vi "Savelot.vi"(5 "Type":string, 7 "Wafer ID":string, 8 "error in (no error)":errorcluster, 11 "LotData in":refnum<class "LotData.lvclass">) -> (0 "error out":errorcluster, 3 "LotData out":refnum<class "LotData.lvclass">)   [LabVIEW 2012, in "LotData.lvclass"]
uses:
  LotData.lvclass
  LotData.lvclass/LotData.ctl
  <vilib>/Utility/file.llb/Read From Spreadsheet File (string).vi
  <vilib>/Utility/file.llb/Write To Spreadsheet File (string).vi
  <vilib>/Utility/file.llb/Write To Spreadsheet File (DBL).vi
panel:
  out "Array":string[][](array[string])
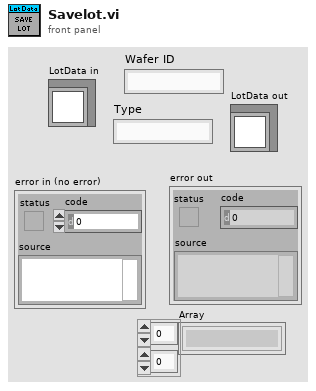
[diagram p1: front panel]
types:
  T1 = cluster{"Area":string, "Wavelength":dbl[], "EL Spectrum":dbl[]}[]
  T2 = typedef "TestData.ctl" = cluster{"20mA Data":cluster{"Area":string, "Current,mA":dbl, "Power":dbl, "WL":dbl, "Voltage":dbl, "Knee Current":dbl, "Reverse":dbl}, "50mA Data":cluster{"Area":string, "Current,mA":dbl, "Power":dbl, "WL":dbl, "Voltage":dbl}}
  T3 = typedef "WaferTable.ctl" = string[][]
  T4 = cluster{"Area":string, "Current,mA":dbl, "Power":dbl, "WL":dbl, "Voltage":dbl, "Knee Current":dbl, "Reverse":dbl}
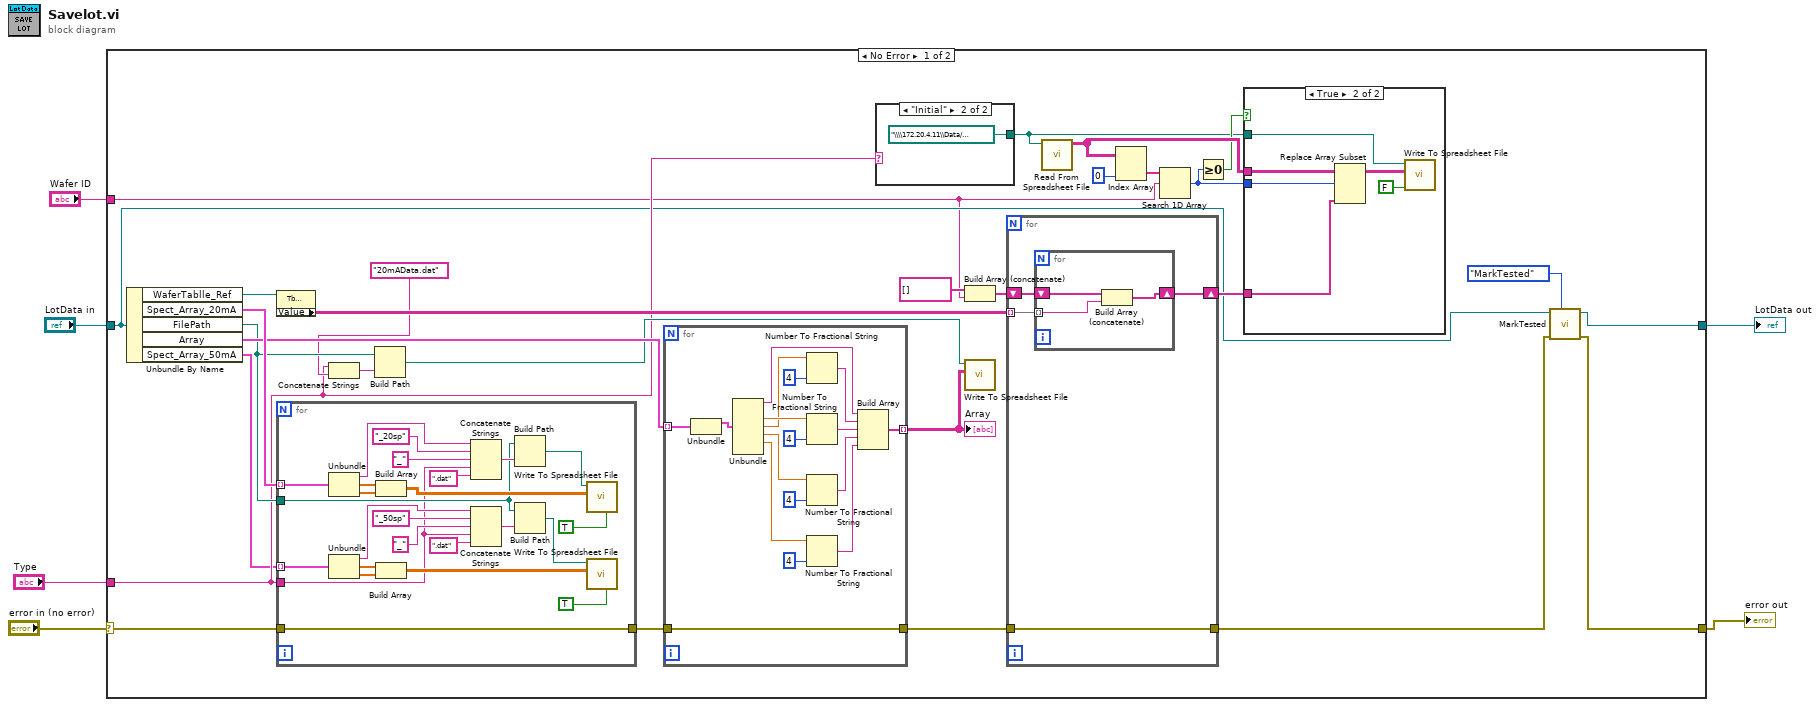
[diagram p0: block diagram]
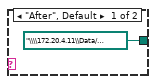
[diagram p2: hidden frame]
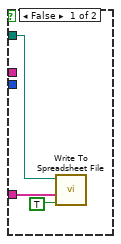
[diagram p3: hidden frame]
diagram:
  n1 = case shown="No Error" "error in (no error)" {
    selector: "error in (no error)" -> [w20 w97]
    tunnel: [w11 w97] -> w1
    tunnel: [w10 w96] -> w4
    tunnel: "LotData in" -> [w9 w96]
    tunnel: "Type" -> [w15 _]
    tunnel: "Wafer ID" -> [w8 _]
    frame No Error {
      n2 = Unbundle By Name(w9) -> ("WaferTablle_Ref"=w35:refnum<vi>, "Spect_Array_20mA"=w24:T1, "FilePath"=w19:path, "Array"=w23:T2[], "Spect_Array_50mA"=w13:T1)
      n3 = property class="Tbl (strict)"(reference=w35) -> ("Value"=w34:T3)  [unwired: 1 in, 2 out]
      n4 = for {
        tunnel: w24 -> [w77] mode=indexing
        tunnel: w19 -> [w54]
        tunnel: w15 -> [w53]
        tunnel: [w67] -> w21
        tunnel: w20 -> [w67]
        tunnel: w13 -> [w55] mode=indexing
        n5 = Unbundle(w77) -> ("Area"=w69:string, "Wavelength"=w73:dbl[], "EL Spectrum"=w72:dbl[])
        n6 = Unbundle(w55) -> ("Area"=w63:string, "Wavelength"=w59:dbl[], "EL Spectrum"=w60:dbl[])
        n7 = Build Array(w73, w72) -> (w71:dbl[][])
        n8 = Build Array(w59, w60) -> (w61:dbl[][])
        n9 = Concatenate Strings(w69, "_20sp" ("string"), "_" ("string"), w53, ".dat" ("string")) -> (w75:string)
        n10 = Concatenate Strings(w63, "_50sp" ("string"), "_" ("string"), w53, ".dat" ("string")) -> (w57:string)
        n11 = Build Path(base path=w54, name or relative path=w75) -> (appended path=w74:path)
        n12 = Build Path(base path=w54, name or relative path=w57) -> (appended path=w58:path)
        n13 = call-poly <vilib>:"Write To Spreadsheet File.vi"("transpose? (no:F)"=TRUE, "2D data"=w71, "file path (dialog if empty)"=w74) -> ()  [unwired: 5 in, 1 out]
        n14 = call-poly <vilib>:"Write To Spreadsheet File.vi"("transpose? (no:F)"=TRUE, "2D data"=w61, "file path (dialog if empty)"=w58) -> ()  [unwired: 5 in, 1 out]
      }
      n15 = Concatenate Strings(w15, "20mAData.dat" ("string")) -> (w14:string)
      n16 = Build Path(base path=w19, name or relative path=w14) -> (appended path=w18:path)
      n17 = for {
        tunnel: w23 -> [w52] mode=indexing
        tunnel: [w41] -> w22
        tunnel: w21 -> [w41]
        tunnel: [w36] -> w17 mode=indexing
        n18 = Unbundle(w52) -> ("20mA Data"=w51:T4)  [unwired: 1 out]
        n19 = Unbundle(w51) -> ("Area"=w37:string, "Power"=w47:dbl, "WL"=w39:dbl, "Voltage"=w46:dbl, "Knee Current"=w45:dbl)  [unwired: 2 out]
        n20 = Number To Fractional String(number=w39, precision (6)=i16 4) -> (F-format string=w38:string)  [unwired: 2 in]
        n21 = Number To Fractional String(number=w47, precision (6)=i16 4) -> (F-format string=w44:string)  [unwired: 2 in]
        n22 = Number To Fractional String(number=w46, precision (6)=i16 4) -> (F-format string=w43:string)  [unwired: 2 in]
        n23 = Number To Fractional String(number=w45, precision (6)=i16 4) -> (F-format string=w42:string)  [unwired: 2 in]
        n24 = Build Array(w37, w38, w44, w43, w42) -> (w36:string[])
      }
      "Array" <- w17
      n25 = case shown="\"Initial\"" w15 {
        tunnel: [path "\\\\172.20.4.11\\Data/Characterization Raw Data/Quick EL Test/Wafer Data_After.dat" ("file path (dialog if empty)") path "\\\\172.20.4.11\\Data/Characterization Raw Data/Quick EL Test/Wafer Data.dat" ("file path (dialog if empty)")] -> w25
        frame "After", Default {
        }
        frame "Initial" {
        }
      }
      n26 = Build Array (concatenate)(string[] [], w8) -> (w32:string[])
      n27 = call-poly <vilib>:"Write To Spreadsheet File.vi"("2D data"=w17, "file path (dialog if empty)"=w18) -> ()  [unwired: 6 in, 1 out]
      n28 = for {
        tunnel: w34 -> [w91] mode=indexing
        shift-right: [w90] -> w26
        shift-left: w32 -> [w92]
        tunnel: [w89] -> w12
        tunnel: w22 -> [w89]
        n29 = for {
          shift-right: [w93] -> w90
          shift-left: w92 -> [w95]
          tunnel: w91 -> [w94] mode=indexing
          n30 = Build Array (concatenate)(w95, w94) -> (w93:string[])
        }
      }
      n31 = call-poly <vilib>:"Read From Spreadsheet File.vi"("file path (dialog if empty)"=w25) -> ("all rows"=w29:string[][])  [unwired: 6 in, 4 out]
      n32 = Index Array(array=w29, index (col)=0 ("index (row)")) -> (element=w30:string[])  [unwired: 1 in]
      n33 = Search 1D Array(1D array=w30, element=w8) -> (index of element=w28:i32)  [unwired: 1 in]
      n34 = Greater Or Equal To 0?(x=w28) -> (x >= 0?=w27:bool)
      n35 = case shown="True" w27 {
        tunnel: w29 -> [_ w86]
        tunnel: w28 -> [_ w85]
        tunnel: w25 -> [w81 w84]
        tunnel: w26 -> [w80 w83]
        frame False {
          n36 = call-poly <vilib>:"Write To Spreadsheet File.vi"("append to file? (new file:F)"=TRUE, "1D data"=w80, "file path (dialog if empty)"=w81) -> ()  [unwired: 5 in, 1 out]
        }
        frame True {
          n37 = Replace Array Subset(array=w86, new element=w83, index (row)=w85) -> (w87:string[][])  [unwired: 1 in]
          n38 = call-poly <vilib>:"Write To Spreadsheet File.vi"("append to file? (new file:F)"=FALSE, "2D data"=w87, "file path (dialog if empty)"=w84) -> ()  [unwired: 5 in, 1 out]
        }
      }
      n39 = call-dynamic "MarkTested.vi"("Enum"=enum16{"MarkTested", "MarkNotTested"}."MarkTested", "error in (no error)"=w12, "LotData in"=w9) -> ("error out"=w11:errorcluster, "LotData out"=w10:refnum<class "LotData.lvclass">)  [unwired: 6 in, 1 out]
    }
    frame Error {
    }
  }
  "error out" <- w1
  "LotData out" <- w4
